vi "Measurement Logic.vi"(8 "error in":errorcluster, 10 "Measurement Context":refnum<class "MeasurementContext.lvclass">, 11 "Measurement Configuration":T3={"Input channel"=0, "Full scale range"=10.0, "Analog source resource name"="", "Frequency"=1000.0, "Amplitude"=-1.0, "Digital capture resource name"="", "Digital capture sample rate"=800000.0, "Digital capture samples"=800000}) -> (0 "error out":errorcluster, 2 "Measurement Context out":refnum<class "MeasurementContext.lvclass">, 3 "Measurement Results":T2)   [LabVIEW 2021, in "ADC_ACMeasurement.lvlib"]
uses:
  adc_acMeasurement.lvlib
  Measurement Configuration.ctl
  Measurement Results.ctl
  <vilib>/MeasurementLink/MeasurementLink Measurement Server/Classes/MeasurementContext/MeasurementContext.lvclass
  <vilib>/gRPC/LabVIEW gRPC Library/Shared/grpcId.ctl
  shared/subVIs/controls/HW Sync Commands.ctl
  <vilib>/DAQmx/create/channels.llb/DAQmx Create Channel (AO-Voltage-Basic).vi
  <vilib>/DAQmx/configure/timing.llb/DAQmx Timing (Sample Clock).vi
  <vilib>/DAQmx/create/channels.llb/DAQmx Create Channel (AO-FuncGen).vi
  <resource>/objmgr/daqmx.rc
  shared/digitalInterface/client/dcvmDPI_AD7606B_client/dcvmDPI_AD7606B_client.lvlib
  shared/digitalInterface/client/dcvmDPI_AD7606B_clientImpl/dcvmDPI_AD7606B_clientImpl.lvlib
  <vilib>/gRPC/LabVIEW gRPC Library/grpc-lvsupport-release.lvlib
panel:
  in  "Pin config":T1(array[cluster])=[{"Pin"="RESET", "Current Limit"=0.01, "Voltage Level"=3.3}, {"Pin"="SCLK", "Current Limit"=0.01, "Voltage Level"=3.3}, {"Pin"="CS", "Current Limit"=0.01, "Voltage Level"=3.3}, {"Pin"="WR", "Current Limit"=0.01, "Voltage Level"=3.3}, {"Pin"="CONVST", "Current Limit"=0.01, "Voltage Level"=0.0}, {"Pin"="REFSEL", "Current Limit"=0.01, "Voltage Level"=3.3}, {"Pin"="STBY", "Current Limit"=0.01, "Voltage Level"=3.3}, {"Pin"="SERPAR", "Current Limit"=0.01, "Voltage Level"=0.0}, {"Pin"="RANGE", "Current Limit"=0.01, "Voltage Level"=0.0}, {"Pin"="OS0", "Current Limit"=0.01, "Voltage Level"=0.0}, {"Pin"="OS1", "Current Limit"=0.01, "Voltage Level"=0.0}, {"Pin"="OS2", "Current Limit"=0.01, "Voltage Level"=0.0}, {"Pin"="RESET", "Current Limit"=0.01, "Voltage Level"=0.0}]
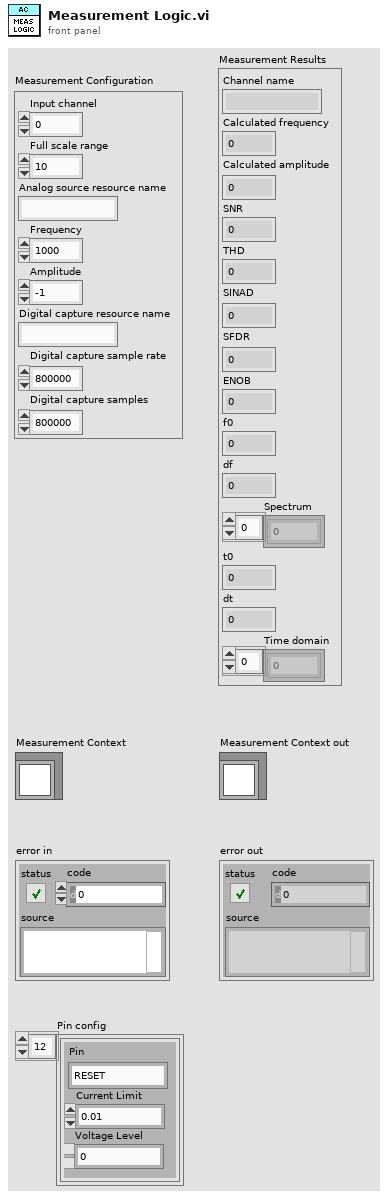
[diagram p1: front panel]
types:
  T1 = cluster{"Pin":string, "Current Limit":dbl, "Voltage Level":dbl}[]
  T2 = typedef "adc_acMeasurement.lvlib/Measurement Results.ctl" = cluster{"Channel name":string, "Calculated frequency":dbl, "Calculated amplitude":dbl, "SNR":dbl, "THD":dbl, "SINAD":dbl, "SFDR":dbl, "ENOB":dbl, "f0":dbl, "df":dbl, "Spectrum":dbl[], "t0":dbl, "dt":dbl, "Time domain":dbl[]}
  T3 = typedef "adc_acMeasurement.lvlib/Measurement Configuration.ctl" = cluster{"Input channel":i32, "Full scale range":dbl, "Analog source resource name":string, "Frequency":dbl, "Amplitude":dbl, "Digital capture resource name":string, "Digital capture sample rate":dbl, "Digital capture samples":u32}
  T4 = typedef "HW Sync Commands.ctl" = enum16{"NoAction", "GenerationStarted", "AcquisitionCompleted", "GenerationErrored"}
  T5 = typedef "grpc-lvsupport-release.lvlib/grpcId.ctl" = u64
  T6 = cluster{"DSG Session":refnum<k21>, "gRPC session":T5}
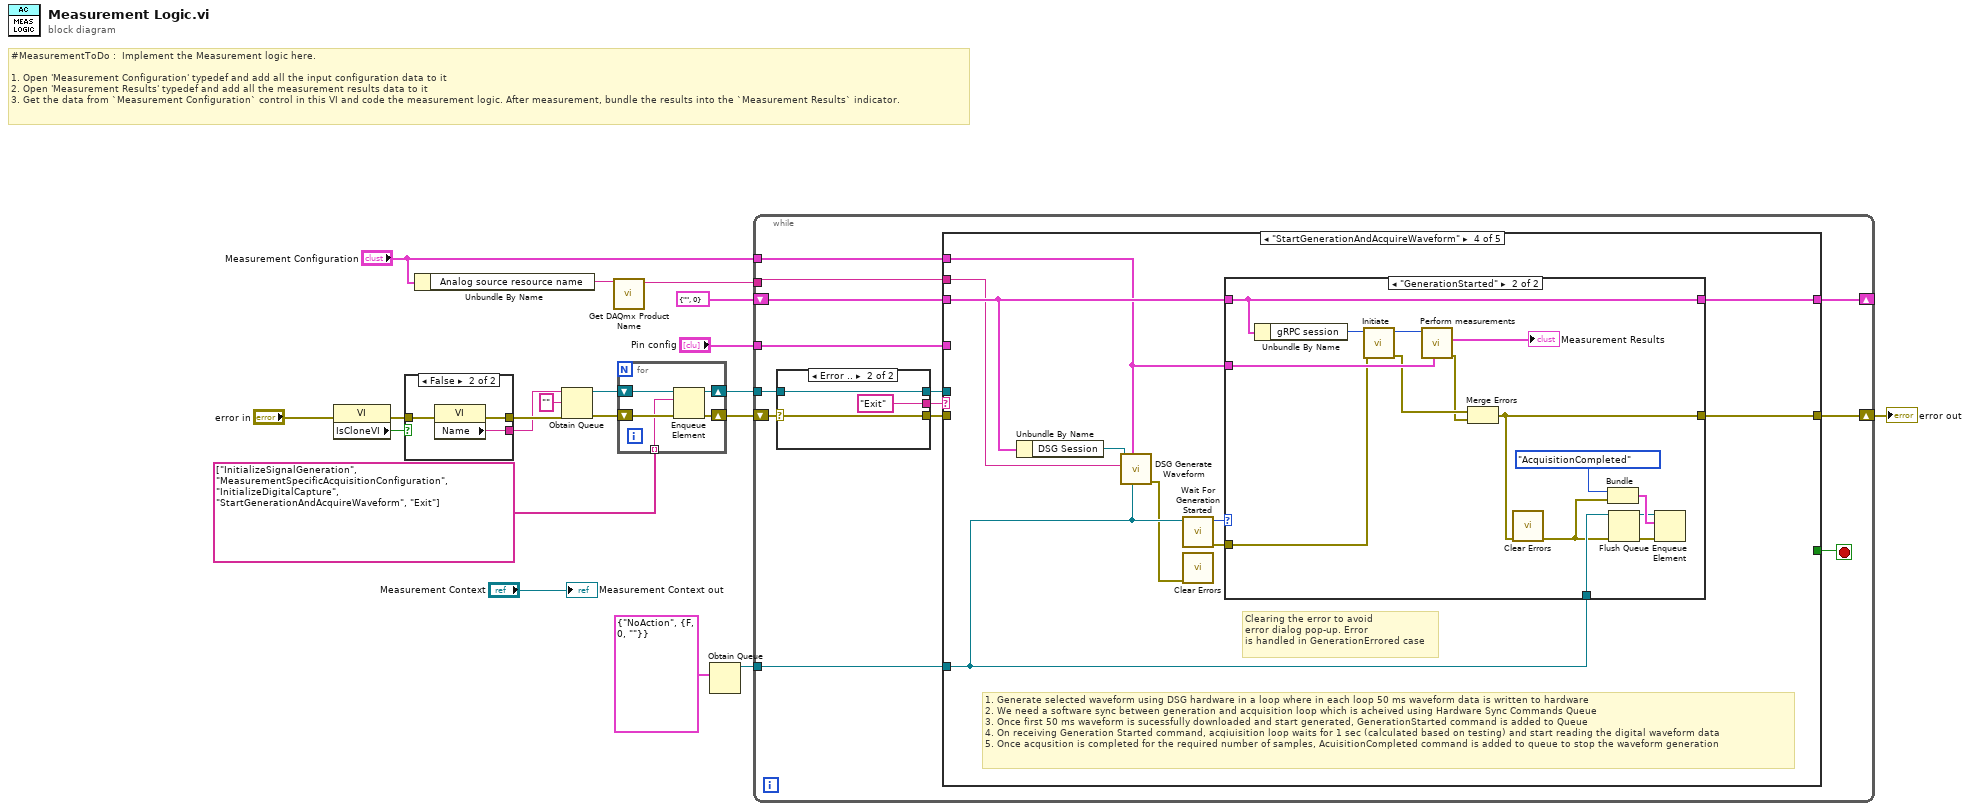
[diagram p0: block diagram]
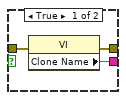
[diagram p2: hidden frame]
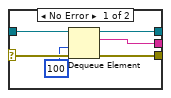
[diagram p3: hidden frame]
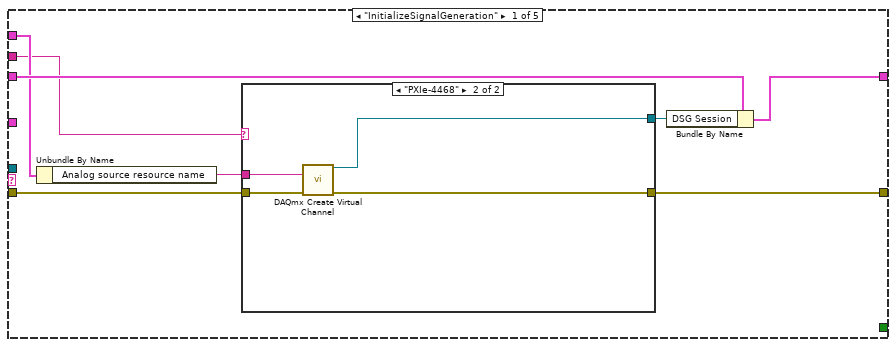
[diagram p4: hidden frame]
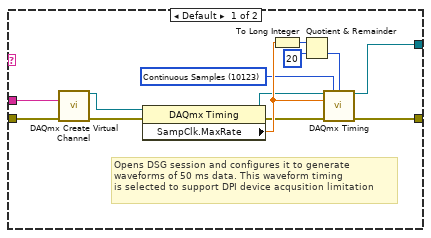
[diagram p5: hidden frame]
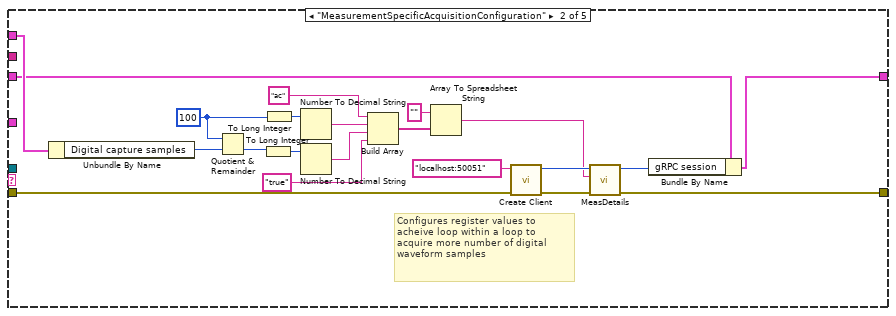
[diagram p6: hidden frame]
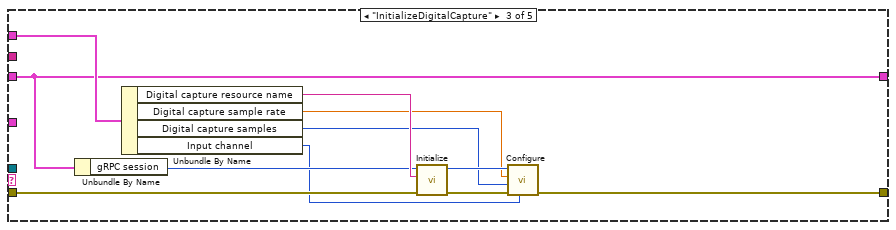
[diagram p7: hidden frame]
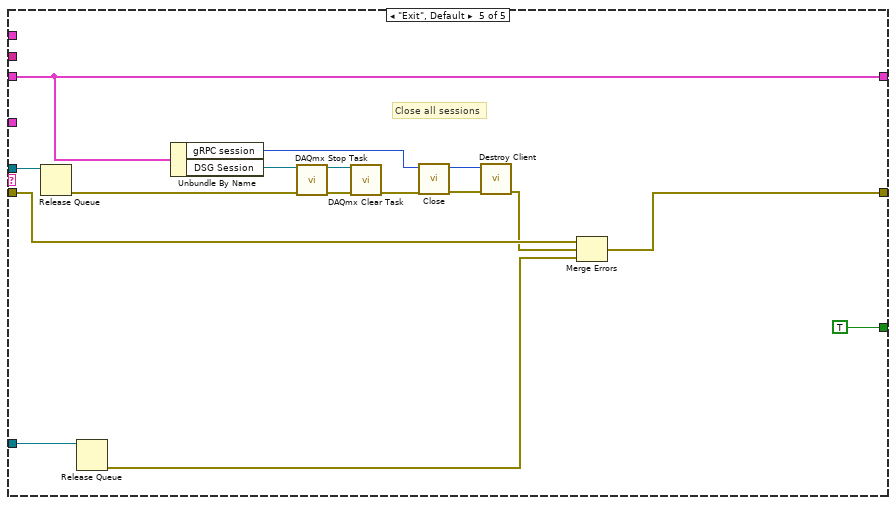
[diagram p9: hidden frame]
diagram:
  # "#MeasurementToDo :  Implement the Measurement logic here.\n\n1. Open 'Measurement Configuration' typedef and add all the input configuration data to it\n2. Open 'Measurement Results' typedef and add all the measurement results data to it\n3. Get the data from `Measurement Configuration` control in this VI and code the measurement logic. After measurement, bundle the results into the `Measurement Results` indicator."
  n1 = property class="VI"(error in="error in") -> (error out=w9:errorcluster, "IsCloneVI"=w10:bool)  [unwired: 1 in, 1 out]
  n2 = case shown="False" w10 {
    tunnel: [w23 w26] -> w7
    tunnel: [w22 w25] -> w6
    tunnel: w9 -> [w21 w24]
    frame True {
      n3 = property class="VI"(error in=w21) -> (error out=w23:errorcluster, "Clone Name"=w22:string)  [unwired: 1 in, 1 out]
    }
    frame False {
      n4 = property class="VI"(error in=w24) -> (error out=w26:errorcluster, "Name"=w25:string)  [unwired: 1 in, 1 out]
    }
  }
  n5 = Unbundle By Name("Measurement Configuration") -> ("Analog source resource name"=w2:string)
  n6 = Obtain Queue(name (unnamed)=w6, element data type="", error in (no error)=w7) -> (queue out=w18:refnum<queue>, error out=w5:errorcluster)  [unwired: 2 in, 1 out]
  n7 = call "Get DAQmx Product Name.vi"("DAQmx resource name"=w2) -> ("DAQmx product type"=w1:string)  [unwired: 10 in]
  n8 = for {
    shift-right: [w29] -> w17
    shift-left: w18 -> [w31]
    shift-right: [w28] -> w4
    shift-left: w5 -> [w30]
    tunnel: string[] ["InitializeSignalGeneration", "MeasurementSpecificAcquisitionConfiguration", "InitializeDigitalCapture", "StartGenerationAndAcquireWaveform", "Exit"] ("Step sequence") -> [w27] mode=indexing
    n9 = Enqueue Element(queue=w31, element=w27, error in (no error)=w30) -> (queue out=w29:refnum<queue>, error out=w28:errorcluster)  [unwired: 1 in, 1 out]
  }
  n10 = Obtain Queue(element data type=cluster{"Status":T4, "Error":errorcluster} {"Status"=enum."NoAction", "Error"={"status"=FALSE, "code"=0, "source"=""}}) -> (queue out=w13:refnum<queue>)  [unwired: 4 in, 2 out]
  n11 = while {
    tunnel: w17 -> [w36]
    shift-right: [w44] -> w11
    shift-left: w4 -> [w37]
    tunnel: "Measurement Configuration" -> [w42]
    shift-right: [w40] -> _
    shift-left: T6 {"DSG Session"="", "gRPC session"=0} ("output cluster") -> [w41]
    tunnel: "Pin config" -> [w39]
    tunnel: w13 -> [w38]
    tunnel: w1 -> [w32]
    stop <- w43 stop-if-true
    n12 = case shown="Error .." w37 {
      selector: w37 -> [w48 w52]
      tunnel: w36 -> [w50 w51]
      tunnel: [w49 "Exit" ("t")] -> w35
      tunnel: [w47 w52] -> w34
      tunnel: [w45 w51] -> w33
      frame No Error {
        n13 = Dequeue Element(queue=w50, timeout in ms (-1)=100, error in (no error)=w48) -> (queue out=w45:refnum<queue>, element=w49:string, error out=w47:errorcluster)  [unwired: 1 out]
      }
      frame Error {
      }
    }
    n14 = case shown="\"StartGenerationAndAcquireWaveform\"" w35 {
      tunnel: [w59 w79 w103 w120 w144] -> w44
      tunnel: w34 -> [w60 w95 w109 _ w145]
      tunnel: [_ _ _ _ TRUE] -> w43
      tunnel: w42 -> [w56 w99 w110 w113 _]
      tunnel: w41 -> [w58 w82 w107 w119 w149]
      tunnel: [w57 w80 w107 w118 w149] -> w40
      tunnel: w39 -> [_ _ _ _ _]
      tunnel: w38 -> [_ _ _ w117 w148]
      tunnel: w33 -> [_ _ _ _ w147]
      tunnel: w32 -> [w54 _ _ w112 _]
      frame "InitializeSignalGeneration" {
        n15 = Unbundle By Name(w56) -> ("Analog source resource name"=w61:string)
        n16 = case shown="\"PXIe-4468\"" w54 {
          tunnel: w61 -> [w74 w75]
          tunnel: w60 -> [w73 w78]
          tunnel: [w72 w77] -> w59
          tunnel: [w62 w76] -> w55
          frame Default {
            w63 = 10123 items=["Finite Samples"=10178, "Continuous Samples"=10123, "Hardware Timed Single Point"=12522] ("sample mode")
            # "Opens DSG session and configures it to generate\nwaveforms of 50 ms data. This waveform timing\nis selected to support DPI device acqusition limitation"
            n17 = call-poly <vilib>:"DAQmx Create Virtual Channel.vi"("physical channels"=w74, "error in"=w73) -> ("task out"=w71:refnum<k21>, "error out"=w70:errorcluster)  [unwired: 12 in]
            n18 = property class="DAQmx Timing"(reference=w71, error in=w70) -> (reference out=w66:refnum<k21>, error out=w67:errorcluster, "SampClk.MaxRate"=w68:dbl)
            n19 = To Long Integer(number=w68) -> (32bit integer=w64:i32)
            n20 = Quotient & Remainder(x=w64, y=20) -> (floor(x/y)=w69:i32)  [unwired: 1 out]
            n21 = call-poly <vilib>:"DAQmx Timing.vi"("task/channels in"=w66, "sample mode"=w63, "samples per channel"=w69, "rate"=w68, "error in"=w67) -> ("task out"=w62:refnum<k21>, "error out"=w72:errorcluster)  [unwired: 9 in]
          }
          frame "PXIe-4468" {
            n22 = call-poly <vilib>:"DAQmx Create Virtual Channel.vi"("physical channels"=w75, "error in"=w78) -> ("task out"=w76:refnum<k21>, "error out"=w77:errorcluster)  [unwired: 12 in]
          }
        }
        n23 = Bundle By Name(cluster=w58, "DSG Session"=w55) -> (w57:T6)
      }
      frame "MeasurementSpecificAcquisitionConfiguration" {
        w96 = u32 100 ("x")
        # "Configures register values to acheive loop within a loop to acquire more number of digital waveform samples"
        n24 = Unbundle By Name(w99) -> ("Digital capture samples"=w98:u32)
        n25 = Quotient & Remainder(x=w96, y=w98) -> (floor(x/y)=w97:u32)  [unwired: 1 out]
        n26 = To Long Integer(number=w97) -> (32bit integer=w91:i32)
        n27 = To Long Integer(number=w96) -> (32bit integer=w92:i32)
        n28 = Number To Decimal String(number=w92) -> (decimal integer string=w88:string)  [unwired: 1 in]
        n29 = Number To Decimal String(number=w91) -> (decimal integer string=w89:string)  [unwired: 1 in]
        n30 = Build Array("ac", w88, w89, "true") -> (w87:string[])
        n31 = Array To Spreadsheet String(array=w87, 3:"" ("format string")) -> (spreadsheet string=w83:string)  [unwired: 1 in]
        n32 = call "Create Client.vi"("error in"=w95, "address"="localhost:50051") -> ("error out"=w84:errorcluster, "gRPC ID Out"=w85:T5)  [unwired: 8 in]
        n33 = call "MeasDetails.vi"("error in"=w84, "Active measurement"=w83, "gRPC session in"=w85) -> ("error out"=w79:errorcluster, "gRPC session out"=w81:T5)  [unwired: 7 in]
        n34 = Bundle By Name(cluster=w82, "gRPC session"=w81) -> (w80:T6)
      }
      frame "InitializeDigitalCapture" {
        n35 = Unbundle By Name(w107) -> ("gRPC session"=w106:T5)
        n36 = Unbundle By Name(w110) -> ("Digital capture resource name"=w108:string, "Digital capture sample rate"=w102:dbl, "Digital capture samples"=w101:u32, "Input channel"=w100:i32)
        n37 = call "Initialize.vi"("error in"=w109, "Digital capture resource name"=w108, "gRPC session in"=w106) -> ("error out"=w104:errorcluster, "gRPC session out"=w105:T5)  [unwired: 7 in]
        n38 = call "Configure.vi"("Input channel"=w100, "error in"=w104, "Digital capture samples"=w101, "Digital capture sample rate"=w102, "gRPC session in"=w105) -> ("error out"=w103:errorcluster)  [unwired: 5 in, 1 out]
      }
      frame "StartGenerationAndAcquireWaveform" {
        # "Clearing the error to avoid\nerror dialog pop-up. Error\nis handled in GenerationErrored case"
        # "1. Generate selected waveform using DSG hardware in a loop where in each loop 50 ms waveform data is written to hardware\n2. We need a software sync between generation and acquisition loop which is acheived using Hardware Sync Commands Queue\n3. Once first 50 ms waveform is sucessfully downloaded and start generated, GenerationStarted command is added to Queue\n4. On receiving Generation Started command, acqiuisition loop waits for 1 sec (calculated based on testing) and start reading the digital waveform data\n5. Once acqusition is completed for the required number of samples, AcuisitionCompleted command is added to queue to stop the waveform generation"
        n39 = Unbundle By Name(w119) -> ("DSG Session"=w111:refnum<k21>)
        n40 = call "DSG Generate Waveform.vi"("hardware commands sync queue"=w117, "measurement configuration"=w113, "DAQmx product name"=w112, "DSG task in"=w111) -> ("error out"=w114:errorcluster)  [unwired: 6 in, 1 out]
        n41 = call "Wait For Generation Started.vi"("hardware commands sync queue"=w117) -> ("error out"=w115:errorcluster, "Status"=w116:T4)  [unwired: 9 in]
        n42 = call <vilib>:"Clear Errors.vi"("error in (no error)"=w114) -> ()  [unwired: 5 in, 2 out]
        n43 = case shown="\"GenerationStarted\"" w116 {
          tunnel: [w121 w125] -> w120
          tunnel: w117 -> [_ w133]
          tunnel: w119 -> [w122 w135]
          tunnel: [w122 w135] -> w118
          tunnel: w113 -> [_ w130]
          tunnel: w115 -> [w121 w126]
          frame Default {
          }
          frame "GenerationStarted" {
            n44 = Unbundle By Name(w135) -> ("gRPC session"=w128:T5)
            n45 = call "Initiate.vi"("error in"=w126, "gRPC session in"=w128) -> ("error out"=w124:errorcluster, "gRPC session out"=w127:T5)  [unwired: 8 in]
            n46 = call "Perform measurements.vi"("measurement configuration"=w130, "gRPC ID Out"=w127) -> ("error out"=w123:errorcluster, "measurement results"=→"Measurement Results":T2)  [unwired: 8 in]
            n47 = Merge Errors(w124, w123) -> (w125:errorcluster)
            n48 = call <vilib>:"Clear Errors.vi"("error in (no error)"=w125) -> ("error out"=w132:errorcluster)  [unwired: 5 in, 1 out]
            n49 = Bundle("element"=HW_Sync_Commands."AcquisitionCompleted", "error out"=w132) -> (w136:cluster{"element":T4, "error out":errorcluster})  [unwired: 1 in]
            n50 = Flush Queue(queue=w133, error in (no error)=w132) -> (queue out=w134:refnum<queue>, error out=w131:errorcluster)  [unwired: 1 out]
            n51 = Enqueue Element(queue=w134, element=w136, error in (no error)=w131) -> ()  [unwired: 1 in, 3 out]
          }
        }
      }
      frame "Exit", Default {
        # "Close all sessions"
        n52 = Release Queue(queue=w147) -> (error out=w146:errorcluster)  [unwired: 2 in, 2 out]
        n53 = Release Queue(queue=w148) -> (error out=w143:errorcluster)  [unwired: 2 in, 2 out]
        n54 = Unbundle By Name(w149) -> ("gRPC session"=w142:T5, "DSG Session"=w152:refnum<k21>)
        n55 = call <vilib>:"DAQmx Stop Task.vi"("task/channels in"=w152, "error in"=w146) -> ("task out"=w151:refnum<k21>, "error out"=w150:errorcluster)  [unwired: 12 in]
        n56 = call <vilib>:"DAQmx Clear Task.vi"("task in"=w151, "error in"=w150) -> ("error out"=w141:errorcluster)  [unwired: 13 in]
        n57 = call "Close.vi"("error in"=w141, "gRPC session in"=w142) -> ("error out"=w140:errorcluster, "gRPC session out"=w139:T5)  [unwired: 8 in]
        n58 = call "Destroy Client.vi"("error in"=w140, "gRPC ID"=w139) -> ("error out"=w138:errorcluster)  [unwired: 9 in]
        n59 = Merge Errors(w145, w138, w143) -> (w144:errorcluster)
      }
    }
  }
  "error out" <- w11
  "Measurement Context out" <- "Measurement Context"
